vi "Host-Top-Level.vi"() -> ()   [LabVIEW 2017]
uses:
  State.ctl
  <vilib>/FPGAPlugInAG/PXIe-6592R/niLvFpga_Open_PXIe-6592R.vi
  <vilib>/rvi/interface/common/dynamic/niFpgaDynamicAddResources.vi
  <vilib>/Utility/error.llb/Error Cluster From Error Code.vi
  <vilib>/rvi/errors/niLvFpgaAdjustHostInterfaceError.vi
  <vilib>/FPGAPlugInAG/Dynamic/niLvFpga_Close_Dynamic.vi
  <vilib>/rvi/interface/nirviOpenFPGA/nirviOpenFPGA.xnode
  FPGA Bitfiles/04lwIpEx_FPGATarget_Fpga-Exercisor-T_x8Gx0i3FMmo.lvbitx
  PXIe-6592/Fpga-Exercisor-Top.vi
  <vilib>/rvi/interface/nirviMethod/nirviMethod.xnode
  <vilib>/rvi/interface/nirviReadWriteControl/nirviReadWriteControl.xnode
  <vilib>/rvi/interface/nirviCloseFPGA/nirviCloseFPGA.xnode
  <vilib>/rvi/errors/niLvFpgaMergeErrorWithErrorCode.vi
  <vilib>/FPGAPlugInAG/Dynamic/niLvFpga_ReadFifo_Dynamic.vi
  <vilib>/rvi/interface/Simulation/niFpgaSimulationCallBeginRW.vi
  <vilib>/FPGAPlugInAG/Dynamic/niLvFpga_WriteFifo_Dynamic.vi
  NiFpgaLv.dll
panel:
  out "AXI_STR_RXD_tready 2":bool
  out "tvalid 2":bool
  out "tdata 2":u32
  out "tlast 2":bool
  out "AXI_STR_RXD_tready_Count 2":u16
  out "tvalid_Count 2":u16
  out "tlast_Count 2":u16
  out "tdata_LastNonZero 2":u32
  out "Read Data 2":u32[](array[numeric]) format="%.0x"
  in  "DataToSend 2":u32[](array[numeric])=[240, 241, 242, 243, 244, 245] format="%.0x"
  in  "Send to FIFO #2":bool
  out "GPO2 Channel 2":u32
  in  "GPO2 Channel 1":u32
  in  "GPIO Write-Read #2":bool
  out "GPO1 Channel 1":u32 format="%.0x"
  out "error out":errorcluster
  out "GPO2 Channel 2":u32 format="%.0x"
  in  "Read all GPO":bool
  out "GPO1 Channel 2":u32
  in  "GPO1 Channel 1":u32
  in  "GPIO Write-Read #1":bool
  out "Read Data":u32[](array[numeric]) format="%.0x"
  in  "DataToSend":u32[](array[numeric])=[240, 241, 242, 243, 244, 245] format="%.0x"
  in  "Send to FIFO #1":bool
  in  "Stop":bool
  in  "error in":errorcluster
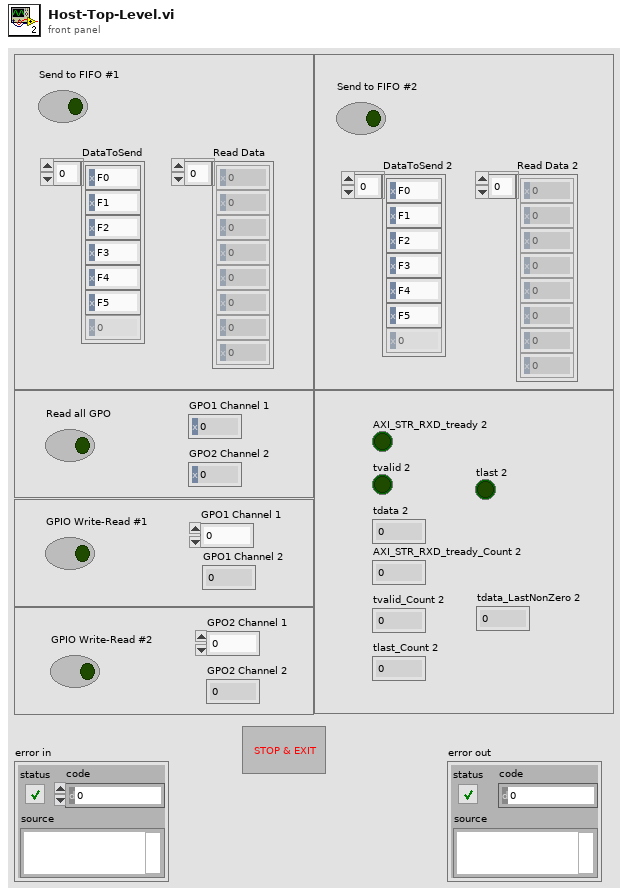
[diagram p1: front panel]
types:
  T1 = typedef "State.ctl" = enum16{"Initialize", "Idle", "Read #1", "Read #2", "Read Status", "Exit"}
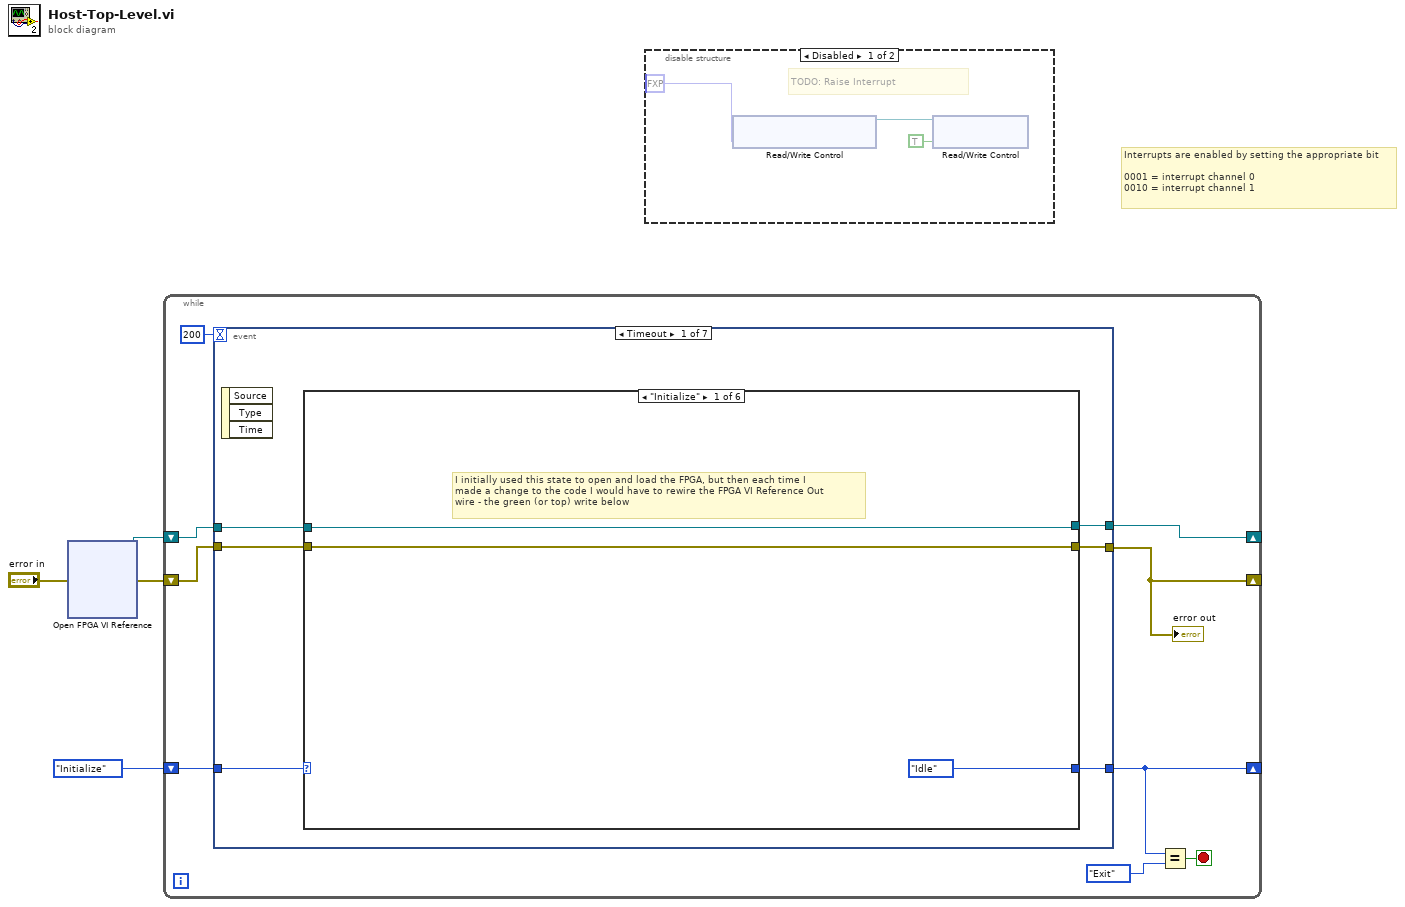
[diagram p0: block diagram]
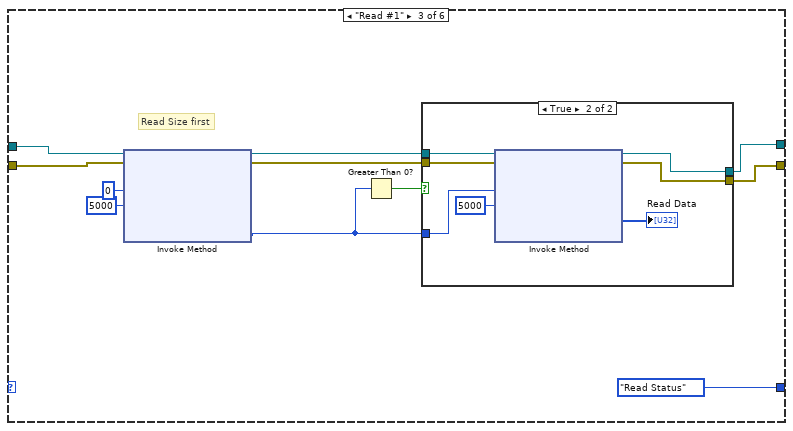
[diagram p4: hidden frame]
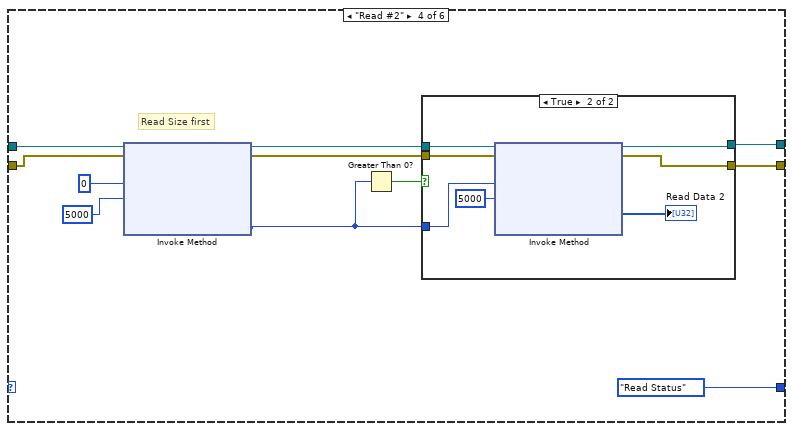
[diagram p6: hidden frame]
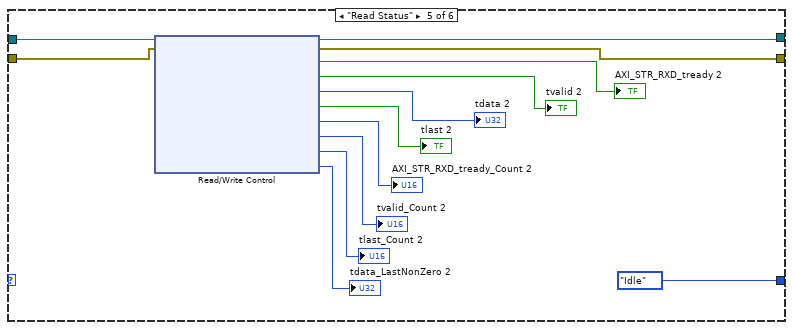
[diagram p8: hidden frame]
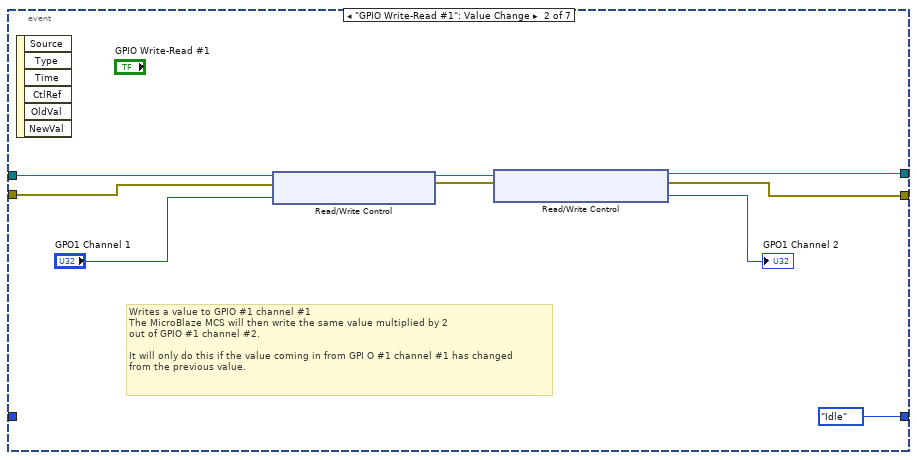
[diagram p10: hidden frame]
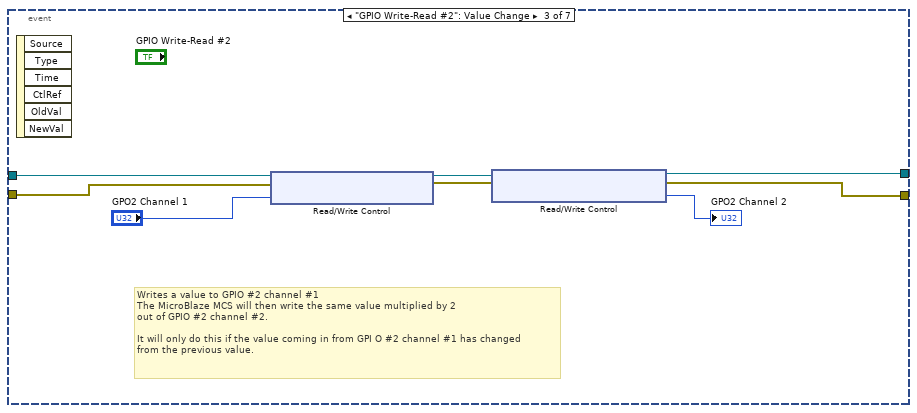
[diagram p11: hidden frame]
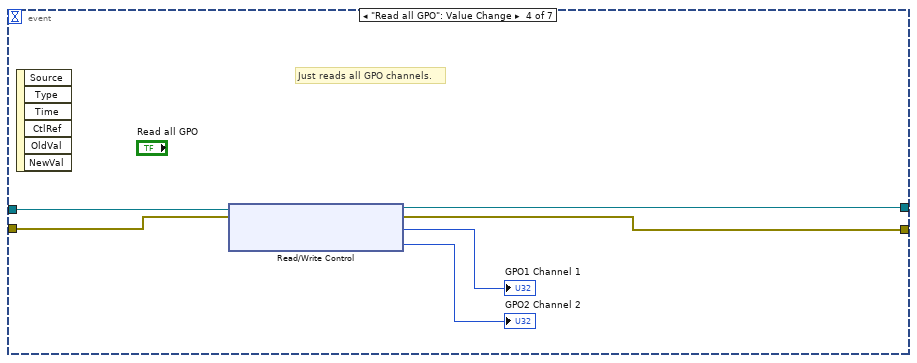
[diagram p12: hidden frame]
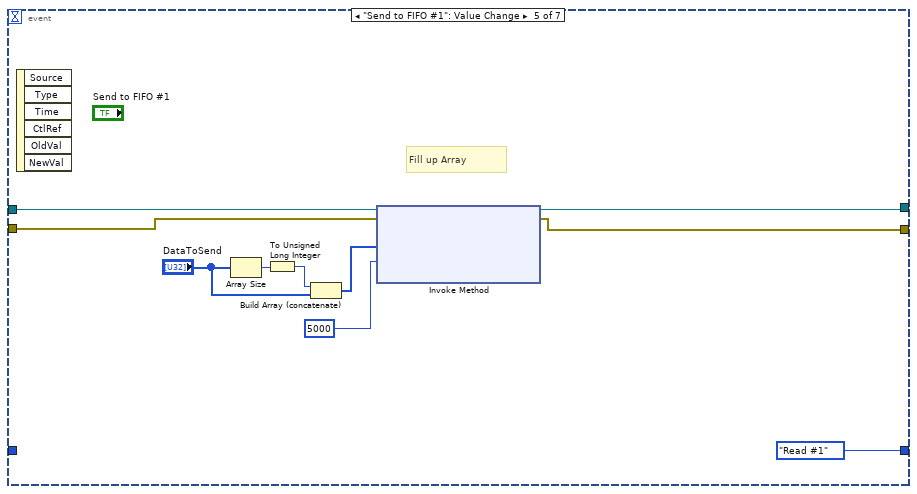
[diagram p13: hidden frame]
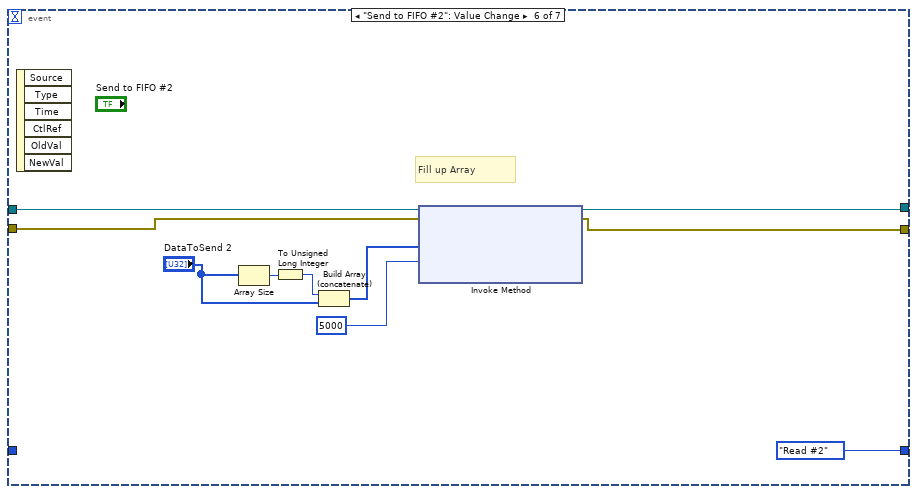
[diagram p14: hidden frame]
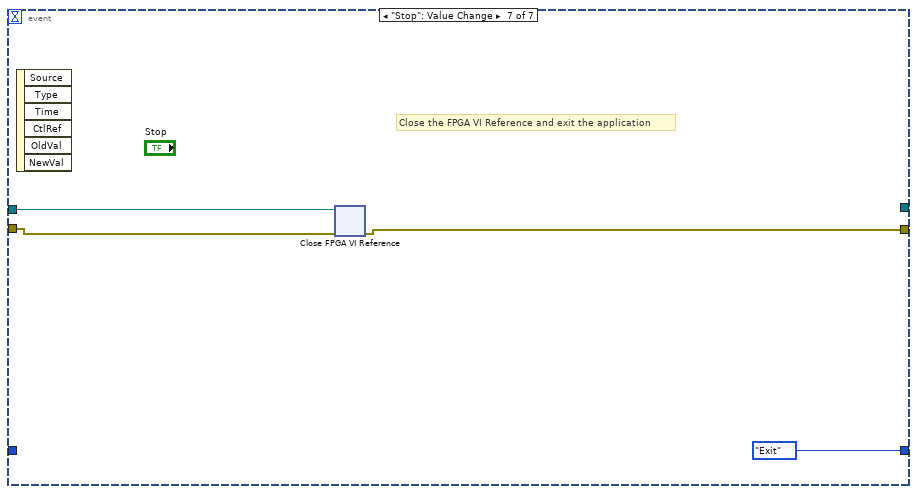
[diagram p15: hidden frame]
diagram:
  # "Interrupts are enabled by setting the appropriate bit\n\n0001 = interrupt channel 0\n0010 = interrupt channel 1"
  n1 = xnode "Open FPGA VI Reference"("error in"="error in") -> ("FPGA VI Reference Out"=w4:refnum<k20>, "error out"=w2:errorcluster)  [unwired: 1 in]
  n2 = while {
    shift-right: [w7] -> _
    shift-left: State."Initialize" ("Enum") -> [w13]
    shift-right: [w8] -> _
    shift-left: w2 -> [w9]
    shift-right: [w6] -> _
    shift-left: w4 -> [w5]
    stop <- w11 stop-if-true
    n3 = event shown="[0] Timeout" {
      selector: _ -> [_ _ _ _ _ _ _]
      dyn-events: _ -> [_ _ _ _ _ _ _]
      timeout: 200 -> [_ _ _ _ _ _ _]
      tunnel: [w17 State."Idle" ("Enum") _ _ State."Read #1" ("Enum") State."Read #2" ("Enum") State."Exit" ("Enum")] -> w7
      tunnel: w13 -> [w16 _ _ _ _ _ _]
      tunnel: w5 -> [w15 w89 w96 w104 w114 w124 w128]
      tunnel: w9 -> [w19 w88 w95 w103 w113 w123 w127]
      tunnel: [w18 w84 w94 w102 w106 w116 w126] -> w8
      tunnel: [w14 w82 w91 w101 w105 w117 _] -> w6
      event Timeout {
        n4 = event-data() -> ()  [unwired: 1 in, 3 out]
        n5 = case shown="\"Initialize\"" w16 {
          selector: w16 -> [_ w24 _ _ _ w80]
          tunnel: w19 -> [w21 w25 w36 w56 w68 w81]
          tunnel: [w21 w25 w31 w51 w67 w81] -> w18
          tunnel: w15 -> [w20 w23 w27 w47 w77 w79]
          tunnel: [State."Idle" ("Enum") w24 State."Read Status" ("Enum") State."Read Status" ("Enum") State."Idle" ("Enum") w80] -> w17
          tunnel: [w20 w23 w28 w48 w66 w79] -> w14
          frame "Initialize" {
            # "I initially used this state to open and load the FPGA, but then each time I \nmade a change to the code I would have to rewire the FPGA VI Reference Out \nwire - the green (or top) write below"
          }
          frame "Idle", Default {
          }
          frame "Read #1" {
            # "Read Size first"
            n6 = xnode "Invoke Method"("FPGA VI Reference In"=w27, "error in"=w36, "Number of Elements"=u32 0, "Timeout (ms)"=5000) -> ("FPGA VI Reference Out"=w32:refnum<k20>, "error out"=w33:errorcluster, "Elements Remaining"=w26:u32)  [unwired: 1 out]
            n7 = Greater Than 0?(x=w26) -> (x > 0?=w29:bool)
            n8 = case shown="True" w29 {
              tunnel: w33 -> [w38 w45]
              tunnel: w32 -> [w37 w44]
              tunnel: [w38 w42] -> w31
              tunnel: [w37 w41] -> w28
              tunnel: w26 -> [_ w39]
              frame False {
              }
              frame True {
                n9 = xnode "Invoke Method"("FPGA VI Reference In"=w44, "error in"=w45, "Number of Elements"=w39, "Timeout (ms)"=5000) -> ("FPGA VI Reference Out"=w41:refnum<k20>, "error out"=w42:errorcluster, "Data"=→"Read Data":u32[])  [unwired: 1 out]
              }
            }
          }
          frame "Read #2" {
            # "Read Size first"
            n10 = xnode "Invoke Method"("FPGA VI Reference In"=w47, "error in"=w56, "Number of Elements"=u32 0, "Timeout (ms)"=5000) -> ("FPGA VI Reference Out"=w52:refnum<k20>, "error out"=w53:errorcluster, "Elements Remaining"=w46:u32)  [unwired: 1 out]
            n11 = Greater Than 0?(x=w46) -> (x > 0?=w49:bool)
            n12 = case shown="True" w49 {
              tunnel: w53 -> [w58 w65]
              tunnel: w52 -> [w57 w64]
              tunnel: [w58 w62] -> w51
              tunnel: [w57 w61] -> w48
              tunnel: w46 -> [_ w60]
              frame False {
              }
              frame True {
                n13 = xnode "Invoke Method"("FPGA VI Reference In"=w64, "error in"=w65, "Number of Elements"=w60, "Timeout (ms)"=5000) -> ("FPGA VI Reference Out"=w61:refnum<k20>, "error out"=w62:errorcluster, "Data"=→"Read Data 2":u32[])  [unwired: 1 out]
              }
            }
          }
          frame "Read Status" {
            n14 = xnode "Read/Write Control"("FPGA VI Reference In"=w77, "error in"=w68) -> ("FPGA VI Reference Out"=w66:refnum<k20>, "error out"=w67:errorcluster, "AXI_STR_RXD_tready"=→"AXI_STR_RXD_tready 2":bool, "tvalid"=→"tvalid 2":bool, "tdata"=→"tdata 2":u32, "tlast"=→"tlast 2":bool, "AXI_STR_RXD_tready_Count"=→"AXI_STR_RXD_tready_Count 2":u16, "tvalid_Count"=→"tvalid_Count 2":u16, "tlast_Count"=→"tlast_Count 2":u16, "tdata_LastNonZero"=→"tdata_LastNonZero 2":u32)
          }
          frame "Exit" {
          }
        }
      }
      event "GPIO Write-Read #1": Value Change {
        # "Writes a value to GPIO #1 channel #1\nThe MicroBlaze MCS will then write the same value multiplied by 2\nout of GPIO #1 channel #2.\n\nIt will only do this if the value coming in from GPI O #1 channel #1 has changed\nfrom the previous value."
        n15 = event-data() -> ()  [unwired: 1 in, 6 out]
        n16 = xnode "Read/Write Control"("FPGA VI Reference In"=w89, "error in"=w88, "d_microblaze\\gpio1_in_tri_i"="GPO1 Channel 1") -> ("FPGA VI Reference Out"=w83:refnum<k20>, "error out"=w86:errorcluster)
        n17 = xnode "Read/Write Control"("FPGA VI Reference In"=w83, "error in"=w86) -> ("FPGA VI Reference Out"=w82:refnum<k20>, "error out"=w84:errorcluster, "d_microblaze\\gpio1_out_tri_o"=→"GPO1 Channel 2":u32)
      }
      event "GPIO Write-Read #2": Value Change {
        # "Writes a value to GPIO #2 channel #1\nThe MicroBlaze MCS will then write the same value multiplied by 2\nout of GPIO #2 channel #2.\n\nIt will only do this if the value coming in from GPI O #2 channel #1 has changed\nfrom the previous value."
        n18 = event-data() -> ()  [unwired: 1 in, 6 out]
        n19 = xnode "Read/Write Control"("FPGA VI Reference In"=w96, "error in"=w95, "d_microblaze\\gpio2_in_tri_i"="GPO2 Channel 1") -> ("FPGA VI Reference Out"=w97:refnum<k20>, "error out"=w98:errorcluster)
        n20 = xnode "Read/Write Control"("FPGA VI Reference In"=w97, "error in"=w98) -> ("FPGA VI Reference Out"=w91:refnum<k20>, "error out"=w94:errorcluster, "d_microblaze\\gpio2_out_tri_o"=→"GPO2 Channel 2":u32)
      }
      event "Read all GPO": Value Change {
        # "Just reads all GPO channels."
        n21 = event-data() -> ()  [unwired: 1 in, 6 out]
        n22 = xnode "Read/Write Control"("FPGA VI Reference In"=w104, "error in"=w103) -> ("FPGA VI Reference Out"=w101:refnum<k20>, "error out"=w102:errorcluster, "d_microblaze\\gpio1_out_tri_o"=→"GPO1 Channel 1":u32, "d_microblaze\\gpio2_out_tri_o"=→"GPO2 Channel 2":u32)
      }
      event "Send to FIFO #1": Value Change {
        # "Fill up Array"
        n23 = event-data() -> ()  [unwired: 1 in, 6 out]
        n24 = Array Size(array="DataToSend") -> (size(s)=w112:i32)
        n25 = To Unsigned Long Integer(number=w112) -> (unsigned 32bit integer=w109:u32)
        n26 = Build Array (concatenate)(w109, "DataToSend") -> (w110:u32[])
        n27 = xnode "Invoke Method"("FPGA VI Reference In"=w114, "error in"=w113, "Data"=w110, "Timeout (ms)"=5000) -> ("FPGA VI Reference Out"=w105:refnum<k20>, "error out"=w106:errorcluster)  [unwired: 1 out]
      }
      event "Send to FIFO #2": Value Change {
        # "Fill up Array"
        n28 = event-data() -> ()  [unwired: 1 in, 6 out]
        n29 = Array Size(array="DataToSend 2") -> (size(s)=w122:i32)
        n30 = To Unsigned Long Integer(number=w122) -> (unsigned 32bit integer=w120:u32)
        n31 = Build Array (concatenate)(w120, "DataToSend 2") -> (w121:u32[])
        n32 = xnode "Invoke Method"("FPGA VI Reference In"=w124, "error in"=w123, "Data"=w121, "Timeout (ms)"=5000) -> ("FPGA VI Reference Out"=w117:refnum<k20>, "error out"=w116:errorcluster)  [unwired: 1 out]
      }
      event "Stop": Value Change {
        # "Close the FPGA VI Reference and exit the application"
        n33 = event-data() -> ()  [unwired: 1 in, 6 out]
        n34 = xnode "Close FPGA VI Reference"("FPGA VI Reference In"=w128, "error in"=w127) -> ("error out"=w126:errorcluster)
      }
    }
    "error out" <- w8
    n35 = Equal?(x=w7, y=State."Exit") -> (x = y?=w11:bool)
  }
  n36 = disable-structure shown="Disabled" {
    frame Disabled {
      # "TODO: Raise Interrupt"
      n37 = xnode "Read/Write Control"("d_mcs_i\\INTC_Interrupt"=fxp<+,4,4> 1.0 ("Interrupt Number")) -> ("FPGA VI Reference In"=w132:refnum<k20>, "FPGA VI Reference Out"=w130:refnum<k20>)  [unwired: 1 in, 1 out]
      n38 = xnode "Read/Write Control"("FPGA VI Reference In"=w130, "Write Interrupt"=TRUE) -> ()  [unwired: 1 in, 2 out]
    }
    frame Enabled {
    }
  }
